vi "SpaceMouse_deadzone.vi"(9 "Space Mouse Input Max":dbl, 10 "Deadzone":dbl, 11 "Filtered Signal":dbl) -> (3 "Deadzoned & Filtered Signal":dbl)   [LabVIEW 2013]
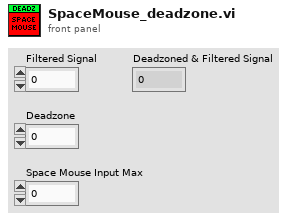
[diagram p1: front panel]
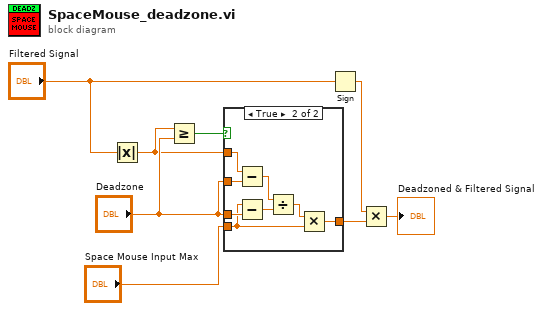
[diagram p0: block diagram]
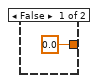
[diagram p2: hidden frame]
diagram:
  n1 = Absolute Value(x="Filtered Signal") -> (abs(x)=w5:dbl)
  n2 = Greater Or Equal?(x=w5, y="Deadzone") -> (x >= y?=w6:bool)
  n3 = case shown="True" w6 {
    tunnel: [0.0 w11] -> w2
    tunnel: w5 -> [_ w16]
    tunnel: "Space Mouse Input Max" -> [_ w10]
    tunnel: "Deadzone" -> [_ w17]
    tunnel: "Deadzone" -> [_ w15]
    frame False {
    }
    frame True {
      n4 = Subtract(x=w16, y=w15) -> (x-y=w14:dbl)
      n5 = Subtract(x=w10, y=w17) -> (x-y=w13:dbl)
      n6 = Divide(x=w14, y=w13) -> (x/y=w12:dbl)
      n7 = Multiply(x=w12, y=w10) -> (x*y=w11:dbl)
    }
  }
  n8 = Sign(1:"Filtered Signal") -> (0:w3:dbl)
  n9 = Multiply(x=w3, y=w2) -> (x*y=→"Deadzoned & Filtered Signal":dbl)
